vi "CRYGet Initialized WFM Array.vi"(0 "Sound Format":T1={"Sample Frequency"=44100.0, "Channels"=2, "bit per sample"=16}, 5 "Time(s)":dbl=0.05, 7 "Rec Padding Time":dbl) -> (4 "initialized array":i32[](array[numeric]), 6 "Time out":dbl=0.05 caption="Record Time(s)", 8 "Record Data Length":u32, 10 "dT":dbl, 14 "real size":i32, 15 "Sample Frequency/2":dbl)   [LabVIEW 2013]
panel:
  in  "Latency (samples)":dbl
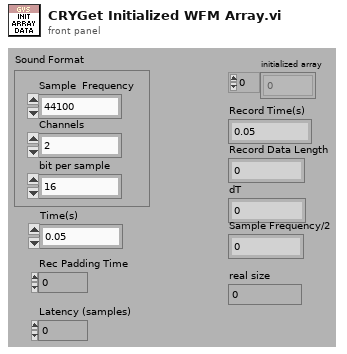
[diagram p1: front panel]
types:
  T1 = cluster{"Sample Frequency":dbl, "Channels":i32, "bit per sample":i32}
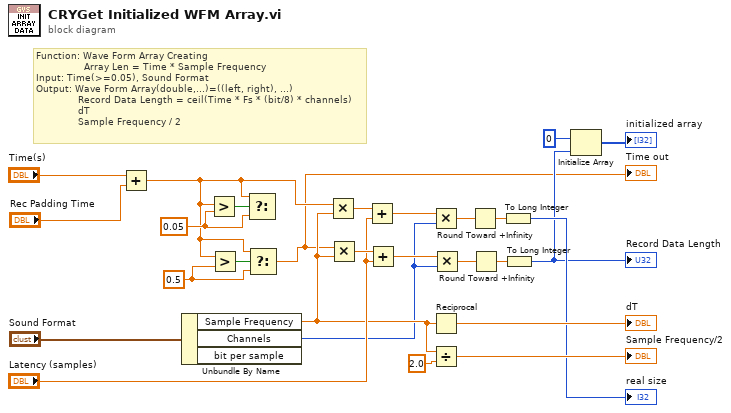
[diagram p0: block diagram]
diagram:
  w5 = 0.5 ("y")
  w13 = 0.05 ("y")
  # "Function: Wave Form Array Creating\n                Array Len = Time * Sample Frequency\nInput: Time(>=0.05), Sound Format\nOutput: Wave Form Array(double,...)=((left, right), ...) \n              Record Data Length = ceil(Time * Fs * (bit/8) * channels)\n              dT\n              Sample Frequency / 2"
  n1 = Add(x="Time(s)", y="Rec Padding Time") -> (x+y=w3:dbl)
  n2 = Unbundle By Name("Sound Format") -> ("Sample Frequency"=w7:dbl, "Channels"=w4:i32)  [unwired: 1 out]
  n3 = Greater?(x=w3, y=w13) -> (0:w22:bool)
  n4 = Greater?(x=w3, y=w5) -> (0:w6:bool)
  n5 = Select(t=w3, s=w22, f=w13) -> ()  [unwired: 1 out]
  n6 = Select(t=w3, s=w6, f=w5) -> (s? t:f=w1:dbl)
  "Time out" <- w1
  n7 = Multiply(x=w3, y=w7) -> (x*y=w15:dbl)
  n8 = Multiply(x=w1, y=w7) -> (x*y=w11:dbl)
  n9 = Add(x=w15, y="Latency (samples)") -> (x+y=w14:dbl)
  n10 = Add(x=w11, y="Latency (samples)") -> (x+y=w12:dbl)
  n11 = Multiply(x=w14, y=w4) -> (x*y=w21:dbl)
  n12 = Reciprocal(x=w7) -> (1/x=→"dT":dbl)
  n13 = Divide(x=w7, y=2.0) -> (x/y=→"Sample Frequency/2":dbl)
  n14 = Multiply(x=w12, y=w4) -> (x*y=w9:dbl)
  n15 = Round Toward +Infinity(x=w21) -> (ceil(x): smallest int >= x=w20:dbl)
  n16 = Round Toward +Infinity(x=w9) -> (ceil(x): smallest int >= x=w10:dbl)
  n17 = To Long Integer(number=w20) -> (32bit integer=→"real size":i32)
  n18 = To Long Integer(number=w10) -> (32bit integer=w2:i32)
  "Record Data Length" <- w2
  n19 = Initialize Array(0 ("element"), w2) -> (→"initialized array":i32[])
